vi "Simple_DAQ_AnalogIO.ProcDestructor.vi"(0 "i ref in":refnum<vi>, 3 "Timeout":i32=10000, 5 "error in":errorcluster caption="Fehler (Eingang, kein Fehler)") -> (14 "i ref out":refnum<vi>, 17 "timed out":bool, 19 "error out":errorcluster caption="Fehler (Ausgang)")   [LabVIEW 2014, in "Simple_DAQ_AnalogIO.lvlib"]
doc: "Contact: Falk Ziegler, info@lab-coding.de"
uses:
  Simple_DAQ_AnalogIO.lvlib
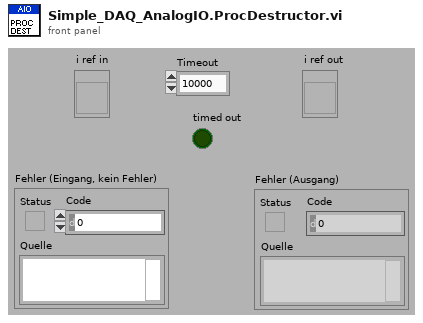
[diagram p1: front panel]
types:
  T1 = typedef "Simple_DAQ_AnalogIO.lvlib/Simple_DAQ_AnalogIO.i attribute.ctl" = cluster{"inputs":cluster{"index":i32[], "channel_task":refnum<k21>[], "range":cluster{"min":dbl, "max":dbl}[], "channel_number":i32, "scale_factor":dbl}, "outputs":cluster{"index":i32[], "channel_task":refnum<k21>[], "range":cluster{"min":dbl, "max":dbl}[], "channel_number":i32, "scale_factor":dbl}}
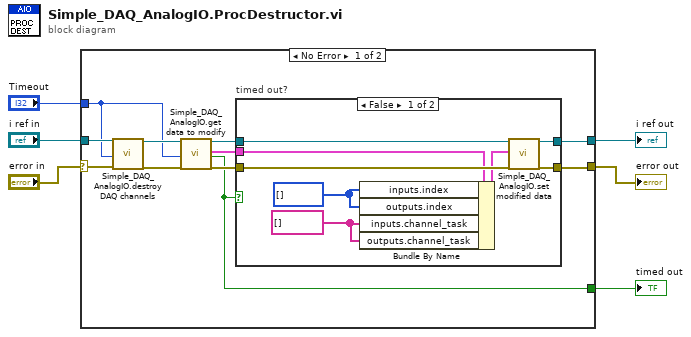
[diagram p0: block diagram]
diagram:
  n1 = case shown="No Error" "error in" {
    selector: "error in" -> [w16 w28]
    tunnel: "i ref in" -> [w17 w29]
    tunnel: [w8 w29] -> w4
    tunnel: [w9 w28] -> w3
    tunnel: "Timeout" -> [w13 _]
    tunnel: [w7 _] -> w1
    frame No Error {
      n2 = call "Simple_DAQ_AnalogIO.destroy DAQ channels.vi"("i ref in"=w17, "Timeout"=w13, "error in"=w16) -> ("i ref out"=w15:refnum<vi>, "error out"=w14:errorcluster)  [unwired: 15 in]
      n3 = call "Simple_DAQ_AnalogIO.get data to modify.vi"("i ref in"=w15, "ms timeout (10000)"=w13, "error in (no error)"=w14) -> ("i ref out"=w11:refnum<vi>, "i attribute"=w10:T1, "timed out"=w7:bool, "error out"=w12:errorcluster)  [unwired: 13 in]
      n4 = case "timed out?" shown="False" w7 {
        tunnel: w12 -> [w24 w26]
        tunnel: w11 -> [w25 w27]
        tunnel: w10 -> [w23 _]
        tunnel: [w21 w26] -> w9
        tunnel: [w20 w27] -> w8
        frame False {
          w18 = string[] []
          w19 = i32[] [] ("Input.nofChannels")
          n5 = Bundle By Name(cluster=w23, "inputs.index"=w19, "outputs.index"=w19, "inputs.channel_task"=w18, "outputs.channel_task"=w18) -> (w22:T1)
          n6 = call "Simple_DAQ_AnalogIO.set modified data.vi"("i ref in"=w25, "i attribute"=w22, "error in (no error)"=w24) -> ("i ref out"=w20:refnum<vi>, "error out"=w21:errorcluster)  [unwired: 15 in]
        }
        frame True {
        }
      }
    }
    frame Error {
    }
  }
  "error out" <- w3
  "timed out" <- w1
  "i ref out" <- w4
